vi "CutSelectRowTable.vi"(8 "エラー入力":errorcluster, 9 "削除する長さ":i32, 10 "削除する指定行":i32, 11 "Tbl refnum":refnum<vi>) -> (0 "エラー出力":errorcluster, 1 "削除部分":string[][](array[string]), 3 "リファレンス出力":refnum<vi>)   [LabVIEW 2014]
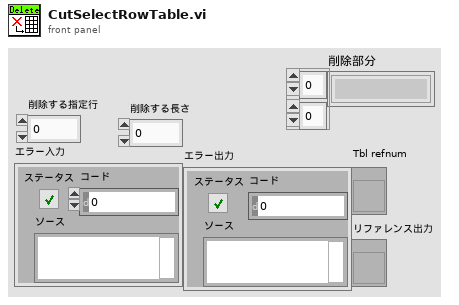
[diagram p1: front panel]
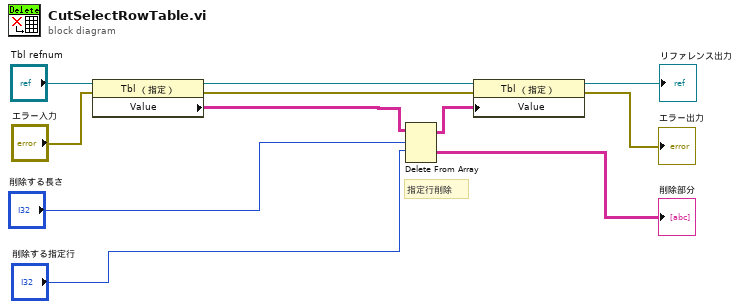
[diagram p0: block diagram]
diagram:
  # "指定行削除"
  n1 = property class="Tbl （指定）"(reference="Tbl refnum", error in="エラー入力") -> (reference out=w7:refnum<vi>, error out=w6:errorcluster, "Value"=w4:string[][])
  n2 = Delete From Array(array=w4, length="削除する長さ", index (row)="削除する指定行") -> (deleted portion=→"削除部分":string[][], array with subset deleted=w5:string[][])  [unwired: 1 in]
  n3 = property class="Tbl （指定）"(reference=w7, error in=w6, "Value"=w5) -> (reference out=→"リファレンス出力":refnum<vi>, error out=→"エラー出力":errorcluster)
